vi "InitBITalino.vi"(6 "Battery \nThreshold (%)":u8(slide)=5 min=5 max=90 step=5 scale=5.0..90.0, 7 "MODE":bool, 8 "error in (no error)":errorcluster, 10 "Sample Rate":enum16{"1", "10", "100", "1000"}(ring), 11 "BITalino":refnum<visa-resource-name>) -> (0 "error out":errorcluster, 2 "Digital Output":bool, 3 "VISA out":refnum<visa-resource-name>)   [LabVIEW 2019]
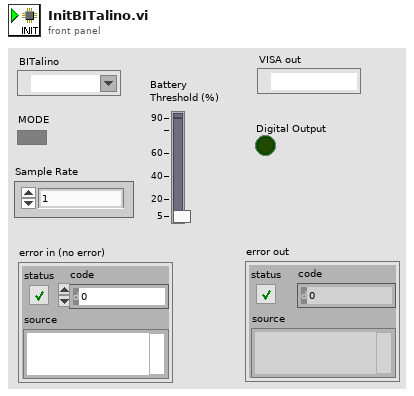
[diagram p1: front panel]
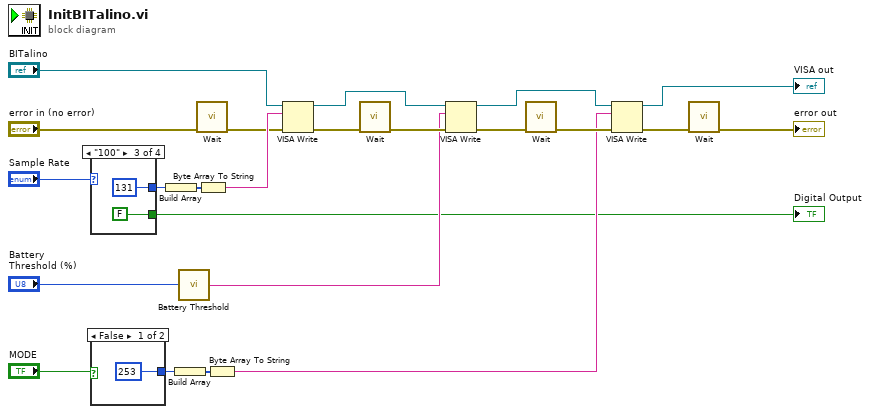
[diagram p0: block diagram]
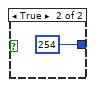
[diagram p2: hidden frame]
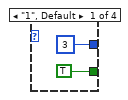
[diagram p3: hidden frame]
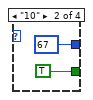
[diagram p4: hidden frame]
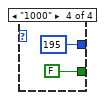
[diagram p5: hidden frame]
diagram:
  n1 = case shown="\"100\"" "Sample Rate" {
    tunnel: [u8 3 u8 67 u8 131 u8 195] -> w21
    tunnel: [TRUE TRUE FALSE FALSE] -> w3
    frame "1", Default {
    }
    frame "10" {
    }
    frame "100" {
    }
    frame "1000" {
    }
  }
  "Digital Output" <- w3
  n2 = case shown="False" "MODE" {
    tunnel: [u8 253 u8 254] -> w16
    frame False {
    }
    frame True {
    }
  }
  n3 = Build Array(w21) -> (w23:u8[])
  n4 = Build Array(w16) -> (w15:u8[])
  n5 = call "Battery Threshold.vi"("Battery \nThreshold (%)"="Battery \nThreshold (%)") -> ("string"=w4:string)
  n6 = call "Wait.vi"("error in (no error)"="error in (no error)") -> ("error out"=w19:errorcluster)  [unwired: 10 in]
  n7 = Byte Array To String(unsigned byte array=w23) -> (string=w20:string)
  n8 = Byte Array To String(unsigned byte array=w15) -> (string=w13:string)
  n9 = VISA Write(VISA resource name="BITalino", write buffer=w20, error in (no error)=w19) -> (VISA resource name out=w7:refnum<visa-resource-name>, error out=w10:errorcluster)  [unwired: 1 out]
  n10 = call "Wait.vi"("error in (no error)"=w10) -> ("error out"=w9:errorcluster)  [unwired: 10 in]
  n11 = VISA Write(VISA resource name=w7, write buffer=w4, error in (no error)=w9) -> (VISA resource name out=w6:refnum<visa-resource-name>, error out=w8:errorcluster)  [unwired: 1 out]
  n12 = call "Wait.vi"("error in (no error)"=w8) -> ("error out"=w18:errorcluster)  [unwired: 10 in]
  n13 = VISA Write(VISA resource name=w6, write buffer=w13, error in (no error)=w18) -> (VISA resource name out=→"VISA out":refnum<visa-resource-name>, error out=w2:errorcluster)  [unwired: 1 out]
  n14 = call "Wait.vi"("error in (no error)"=w2) -> ("error out"=→"error out":errorcluster)  [unwired: 10 in]
